vi "listdir.vi"() -> ()   [LabVIEW 2012]
uses:
  <vilib>/addons/internet/NI_InternetTK_Core_VIs.lvlib
panel:
  out "HTML out":string
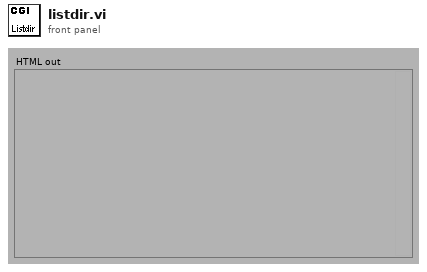
[diagram p1: front panel]
types:
  T1 = typedef "CGI Connection Info.ctl" = cluster{"name":string, "type":T2, "session":T3}
  T2 = typedef "CGI Request Type.ctl" = enum16{"cgi", ".spool first", ".spool", ".spool last"}
  T3 = typedef "HTTP Session.ctl" = refnum<k1>
  T4 = typedef "NI_FTP.lvlib/Keyed Array.ctl" = cluster{"keys":string[], "values":string[]}
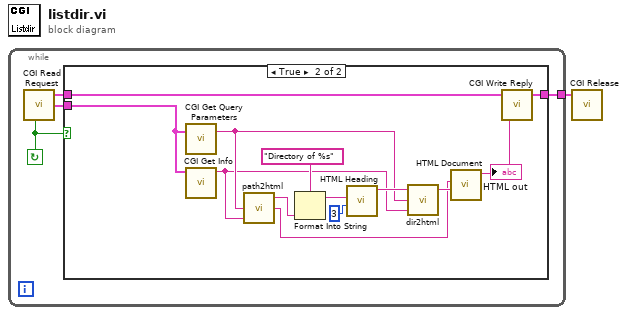
[diagram p0: block diagram]
diagram:
  n1 = while {
    tunnel: [w4] -> w1
    stop <- w2 continue-if-true
    n2 = call <vilib>:"CGI Read Request.vi"() -> ("valid request?"=w2:bool, "cgi connection info"=w5:T1, "env"=w3:T4)  [unwired: 4 in, 1 out]
    n3 = case shown="True" w2 {
      tunnel: [w6 w19] -> w4
      tunnel: w5 -> [w6 w18]
      tunnel: w3 -> [_ w9]
      frame False {
      }
      frame True {
        n4 = call <vilib>:"CGI Get Query Parameters.vi"("env"=w9) -> ("query string"=w8:string)  [unwired: 2 out]
        n5 = call <vilib>:"CGI Get Info.vi"("env"=w9) -> ("cgi name"=w7:string)  [unwired: 4 in, 2 out]
        n6 = call "path2html.vi"("self"=w7, "dir"=w8) -> ("title"=w13:string, "html out"=w16:string)  [unwired: 2 in]
        n7 = Format Into String(format string="Directory of %s", w16) -> (resulting string=w12:string)  [unwired: 2 in, 1 out]
        n8 = call <vilib>:"HTML Heading.vi"("level (1)"=3, "heading"=w12) -> ("HTML out"=w11:string)  [unwired: 9 in]
        n9 = call "dir2html.vi"("self"=w7, "dir"=w8, "html in"=w11) -> ("html out"=w14:string)  [unwired: 2 in]
        n10 = call <vilib>:"HTML Document.vi"("document body"=w14, "document title"=w13) -> ("HTML Document"=w15:string)  [unwired: 9 in]
        "HTML out" <- w15
        n11 = call <vilib>:"CGI Write Reply.vi"("content"=w15, "cgi connection info"=w18) -> ("cgi connection info out"=w19:T1)  [unwired: 3 in]
      }
    }
  }
  n12 = call <vilib>:"CGI Release.vi"("cgi connection info"=w1) -> ()  [unwired: 5 in]
